vi "Highlight Object.vi"(8 "Error In":errorcluster, 10 "Tag":string, 11 "Bookmarks":T1[](array[typedef])) -> (0 "Error Out":errorcluster)   [LabVIEW 2017, in "Bookmark Manager.lvlib"]
uses:
  Bookmark Manager.lvlib
  Controls/VI Bookmark.ctl
  Controls/VI Information.ctl
  Controls/Application Information.ctl
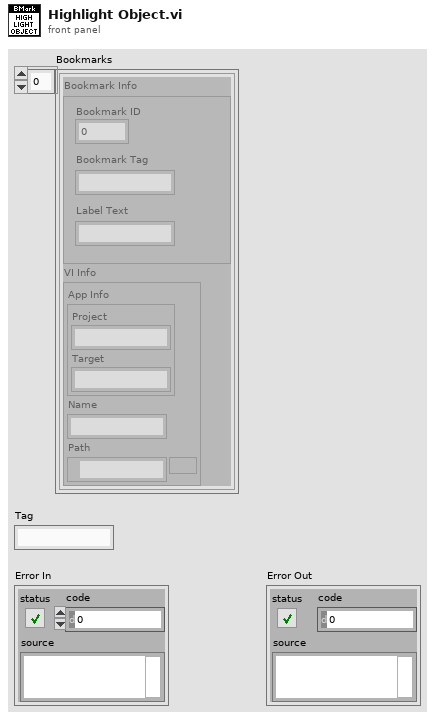
[diagram p1: front panel]
types:
  T1 = typedef "Bookmark Manager.lvlib/VI Bookmark.ctl" = cluster{"Bookmark Info":cluster{"Bookmark ID":u32, "Bookmark Tag":string, "Label Text":string}, "VI Info":T2}
  T2 = typedef "Bookmark Manager.lvlib/VI Information.ctl" = cluster{"App Info":T3, "Name":string, "Path":path}
  T3 = typedef "Bookmark Manager.lvlib/Application Information.ctl" = cluster{"Project":string, "Target":string}
  T4 = enum32{"Bad", "Idle", "Run top level", "Running"}
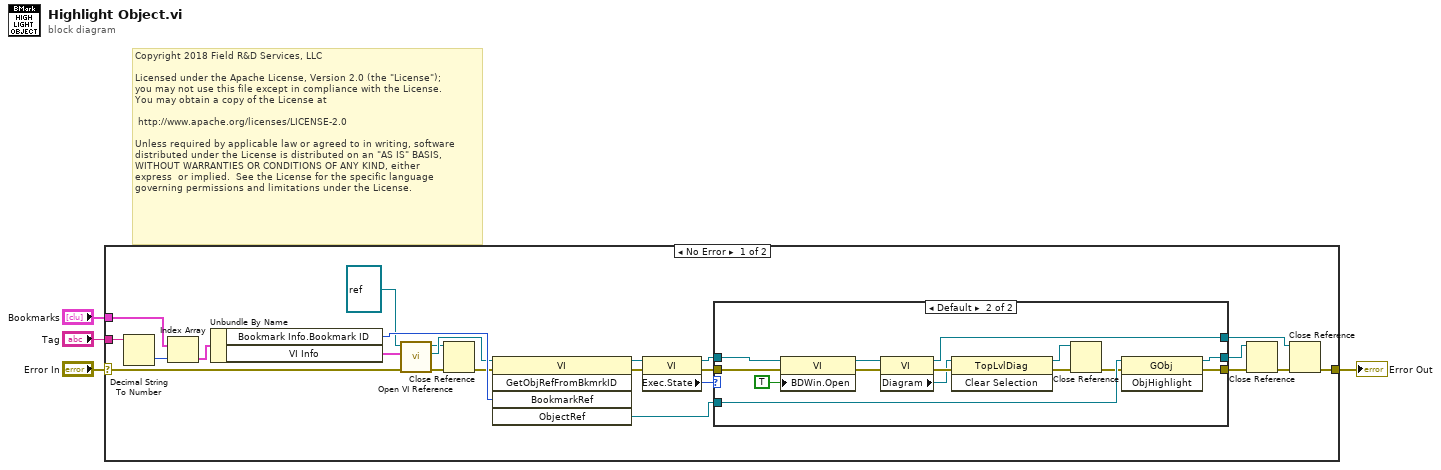
[diagram p0: block diagram]
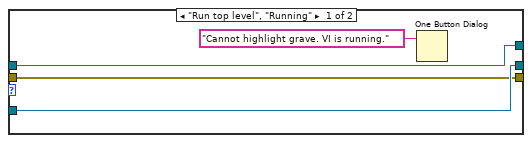
[diagram p2: hidden frame]
diagram:
  # "Copyright 2018 Field R&D Services, LLC\n\nLicensed under the Apache License, Version 2.0 (the \"License\");\nyou may not use this file except in compliance with the License.\nYou may obtain a copy of the License at\n\n\thttp://www.apache.org/licenses/LICENSE-2.0\n\nUnless required by applicable law or agreed to in writing, software\ndistributed under the License is distributed on an \"AS IS\" BASIS,\nWITHOUT WARRANTIES OR CONDITIONS OF ANY KIND, either \nexpress  or implied.  See the License for the specific language \ngoverning permissions and limitations under the License."
  n1 = case shown="No Error" "Error In" {
    selector: "Error In" -> [w12 w46]
    tunnel: [w27 w46] -> w4
    tunnel: "Bookmarks" -> [w25 _]
    tunnel: "Tag" -> [w26 _]
    frame No Error {
      n2 = Decimal String To Number(string=w26) -> (number=w24:i32)  [unwired: 2 in, 1 out]
      n3 = Index Array(array=w25, index=w24) -> (element=w23:T1)
      n4 = Unbundle By Name(w23) -> ("Bookmark Info.Bookmark ID"=w10:u32, "VI Info"=w9:T2)
      n5 = call "Open VI Reference.vi"("Error In"=w12, "VI Info"=w9, "App In"=refnum<vi> refnum) -> ("Error Out"=w11:errorcluster, "VI"=w8:refnum<vi>, "App Out"=w6:refnum<vi>)  [unwired: 6 in]
      n6 = Close Reference(reference=w6, error in (no error)=w11) -> (error out=w7:errorcluster)
      n7 = invoke class="VI" method="GetObjRefFromBkmrkID"(reference=w8, error in=w7, "BookmarkRef"=w10) -> (reference out=w21:refnum<vi>, error out=w22:errorcluster, "ObjectRef"=w17:refnum<vi>)  [unwired: 2 in, 2 out]
      n8 = property class="VI"(reference=w21, error in=w22) -> (reference out=w16:refnum<vi>, error out=w19:errorcluster, "Exec.State"=w20:T4)
      n9 = case shown="Default" w20 {
        tunnel: [w29 w42] -> w18
        tunnel: w19 -> [w29 w38]
        tunnel: w17 -> [w30 w45]
        tunnel: w16 -> [w31 w43]
        tunnel: [w31 w32] -> w15
        tunnel: [w30 w44] -> w13
        frame "Run top level", "Running" {
          n10 = One Button Dialog(message="Cannot highlight grave. VI is running.") -> ()  [unwired: 1 in, 1 out]
        }
        frame Default {
          n11 = property class="VI"(reference=w43, error in=w38, "BDWin.Open"=TRUE ("Block Diagram Window:Open")) -> (reference out=w39:refnum<vi>, error out=w37:errorcluster)
          n12 = property class="VI"(reference=w39, error in=w37) -> (reference out=w32:refnum<vi>, error out=w41:errorcluster, "Diagram"=w40:refnum<vi>)
          n13 = invoke class="TopLvlDiag" method="Clear Selection"(reference=w40, error in=w41) -> (reference out=w35:refnum<vi>, error out=w34:errorcluster)  [unwired: 1 in, 1 out]
          n14 = Close Reference(reference=w35, error in (no error)=w34) -> (error out=w33:errorcluster)
          n15 = invoke class="GObj" method="ObjHighlight"(reference=w45, error in=w33) -> (reference out=w44:refnum<vi>, error out=w42:errorcluster)  [unwired: 1 in, 1 out]
        }
      }
      n16 = Close Reference(reference=w13, error in (no error)=w18) -> (error out=w14:errorcluster)
      n17 = Close Reference(reference=w15, error in (no error)=w14) -> (error out=w27:errorcluster)
    }
    frame Error {
    }
  }
  "Error Out" <- w4
